vi "Initialize Sessions.vi"   [LabVIEW 2021, in "Session Management niSwitch.lvlib"]
doc: "Create the NI-Switch driver session(s) from a reservation."
uses:
  Session Management niSwitch.lvlib
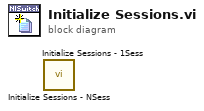
[diagram p0: block diagram]
diagram:
  n1 = call "Initialize Sessions - NSess.vi"() -> ()  [unwired: 8 in, 4 out]
  n2 = call "Initialize Sessions - 1Sess.vi"() -> ()  [unwired: 8 in, 4 out]
